vi "Filter by Message.vi"(10 "Message":string, 11 "Chronological List in":refnum<class "Chronological List.lvclass">) -> (2 "Include?":bool, 3 "Chronological List out":refnum<class "Chronological List.lvclass">)   [LabVIEW 2020, in "Chronological List.lvclass"]
uses:
  Chronological List.lvclass
  Chronological List.lvclass/Chronological List.ctl
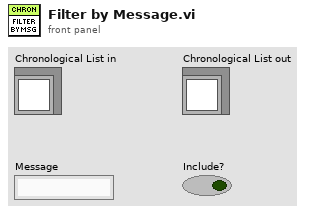
[diagram p1: front panel]
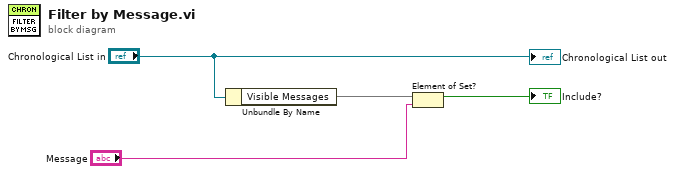
[diagram p0: block diagram]
diagram:
  n1 = Unbundle By Name("Chronological List in") -> ("Visible Messages"=w3:set{string})
  n2 = Element of Set?(10:"Message", 11:w3) -> (3:→"Include?":bool)
  "Chronological List out" <- "Chronological List in"
